vi "Go.vi"(9 "Timing Values":dbl[](array[numeric]), 10 "Control In":T1, 11 "CAD Dispense in":refnum<class "CAD Dispense.lvclass">) -> (2 "Control Out":T1, 3 "CAD Dispense Out":refnum<class "CAD Dispense.lvclass">)   [LabVIEW 2019, in "CAD Dispense.lvclass"]
uses:
  CAD Dispense.lvclass
  Controller/Controllers.ctl
  Controller/I-O/I-O.lvclass
  Controller/Dispenser/Dispenser.lvclass
  C:/Program Files (x86)/Aerotech/A3200/LabVIEW/2010/Bin/Aerotech.A3200.dll
  Program Files (x86)/Aerotech/A3200/LabVIEW/2010/Bin/Aerotech.A3200.dll
  CAD Dispense.lvclass/CAD Dispense.ctl
  Controller/Motion/A3200/A3200.lvclass
  Controller/Controller.lvclass
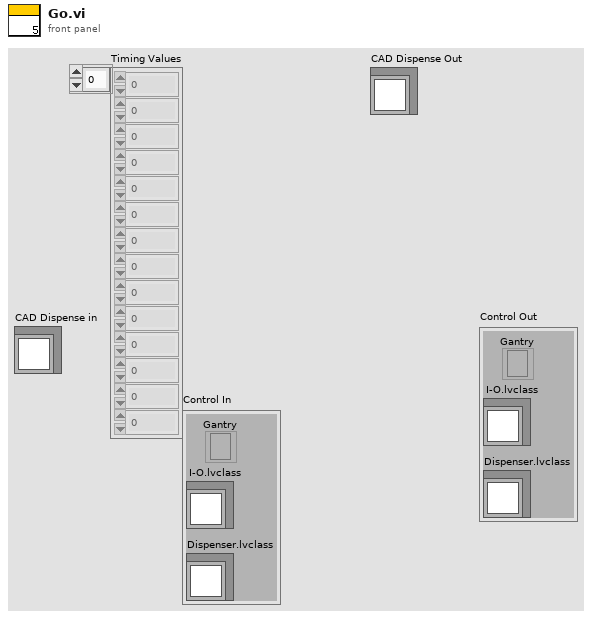
[diagram p1: front panel]
types:
  T1 = typedef "Controller.lvclass/Controllers.ctl" = cluster{"I-O.lvclass":refnum<class "I-O.lvclass">, "Dispenser.lvclass":refnum<class "Dispenser.lvclass">, "Gantry":refnum<k24>}
  T2 = cluster{"Motion":dbl[][], "Center":dbl[], "Circle?":bool, "CW/CCW":dbl}[]
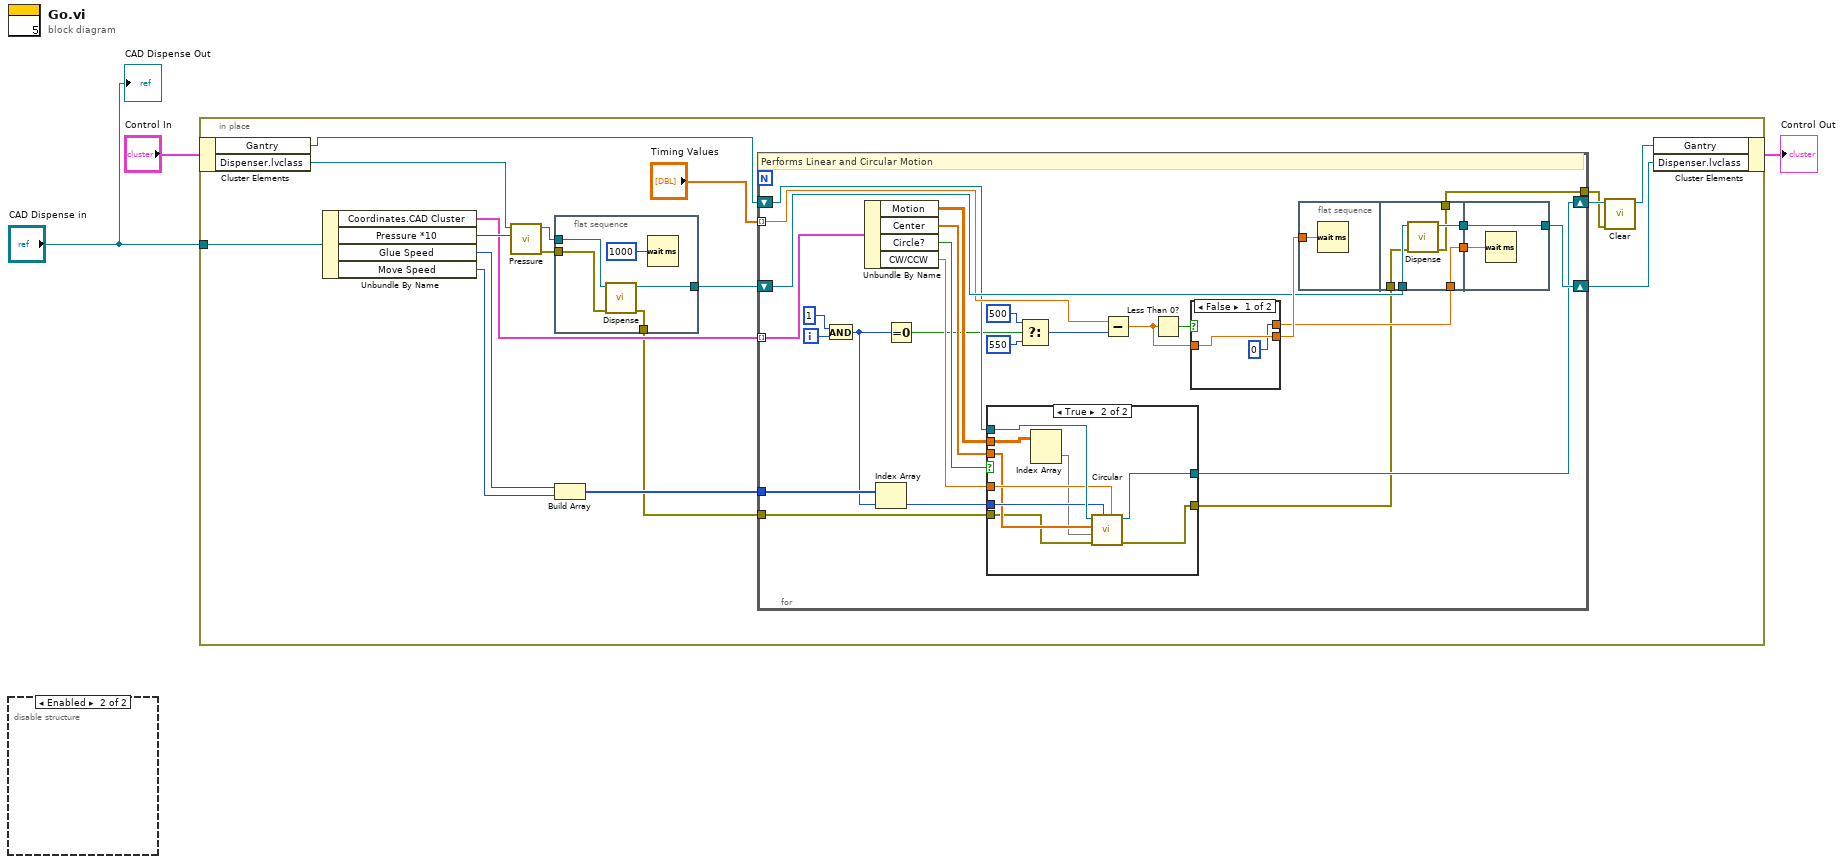
[diagram p0: block diagram]
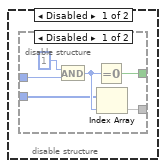
[diagram p2: hidden frame]
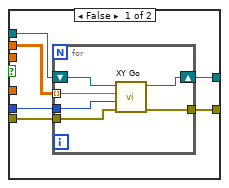
[diagram p4: hidden frame]
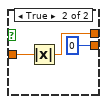
[diagram p5: hidden frame]
diagram:
  n1 = disable-structure shown="Enabled" {
    frame Disabled {
      n2 = disable-structure shown="Disabled" {
        disable-tunnel: [w8 _] -> _
        disable-tunnel: _ -> [w7 _]
        disable-tunnel: [w5 _] -> _
        disable-tunnel: _ -> [w4 _]
        frame Disabled {
          n3 = And(x=1, y=w7) -> (x .and. y?=w6:i32)
          n4 = Equal To 0?(x=w6) -> (x = 0?=w5:bool)
          n5 = Index Array(array=w4, index=w6) -> (element=w8)
        }
        frame Enabled {
        }
      }
    }
    frame Enabled {
    }
  }
  n6 = in-place {
    in-place-border: "CAD Dispense in" -> [w25]
    n7 = in-place-cluster #1("Control In") -> ("Gantry"=w19:refnum<k24>, "Dispenser.lvclass"=w16:refnum<class "Dispenser.lvclass">)
    n8 = Unbundle By Name(w25) -> ("Coordinates.CAD Cluster"=w12:T2, "Pressure *10"=w15:i64, "Glue Speed"=w23:i32, "Move Speed"=w22:i32)
    n9 = call-dynamic "Pressure.vi"("Pressure"=w15, "Dispenser in"=w16) -> ("error out"=w14:errorcluster, "Dispenser out"=w13:refnum<class "Dispenser.lvclass">)  [unwired: 8 in]
    n10 = flat-sequence {
      tunnel: [w29] -> w24
      tunnel: w14 -> [w28]
      tunnel: w13 -> [w30]
      tunnel: [w27] -> w11
      frame #0 {
        n11 = call-dynamic "Dispense.vi"("error in (no error)"=w28, "Dispenser in"=w30) -> ("error out"=w27:errorcluster, "Dispenser out"=w29:refnum<class "Dispenser.lvclass">)  [unwired: 8 in]
        n12 = Wait (ms)(milliseconds to wait=u32 1000) -> ()  [unwired: 1 out]
      }
    }
    n13 = Build Array(w23, w22) -> (w21:i32[])
    n14 = for {
      tunnel: w12 -> [w52] mode=indexing
      tunnel: "Timing Values" -> [w48] mode=indexing
      tunnel: w21 -> [w42]
      shift-right: [w45] -> w26
      shift-left: w24 -> [w54]
      shift-right: [w44] -> w18
      shift-left: w19 -> [w47]
      tunnel: w11 -> [w34]
      tunnel: [w32] -> w10
      i -> [w41]
      # "Performs Linear and Circular Motion"
      n15 = And(x=1, y=w41) -> (x .and. y?=w39:i32)
      n16 = Unbundle By Name(w52) -> ("Motion"=w51:dbl[][], "Center"=w50:dbl[], "Circle?"=w43:bool, "CW/CCW"=w46:dbl)
      n17 = Index Array(array=w42, index=w39) -> (element=w35:i32)
      n18 = Equal To 0?(x=w39) -> (x = 0?=w38:bool)
      n19 = case shown="True" w43 {
        tunnel: [w65 w78] -> w44
        tunnel: w46 -> [_ w76]
        tunnel: w51 -> [w63 w80]
        tunnel: w50 -> [_ w75]
        tunnel: w47 -> [w64 w79]
        tunnel: w35 -> [w62 w77]
        tunnel: w34 -> [w61 w73]
        tunnel: [w60 w72] -> w33
        frame False {
          n20 = for {
            tunnel: w63 -> [w69] mode=indexing
            shift-right: [w70] -> w65
            shift-left: w64 -> [w71]
            tunnel: w62 -> [w68]
            tunnel: w61 -> [w67]
            tunnel: [w66] -> w60
            n21 = call "XY Go.vi"("error in (no error)"=w67, "Speed"=w68, "XY"=w69, "Gantry In"=w71) -> ("error out"=w66:errorcluster, "Gantry Out"=w70:refnum<k24>)  [unwired: 6 in]
          }
        }
        frame True {
          n22 = Index Array(array=w80) -> (element=w74:dbl[])  [unwired: 2 in]
          n23 = call "Circular.vi"("Direction"=w76, "Speed"=w77, "error in (no error)"=w73, "XY End"=w74, "XY Center"=w75, "Gantry In"=w79) -> ("error out"=w72:errorcluster, "Gantry Out"=w78:refnum<k24>)  [unwired: 4 in]
        }
      }
      n24 = Select(t=500, s=w38, f=550) -> (s? t:f=w53:i32)
      n25 = Subtract(x=w48, y=w53) -> (x-y=w49:dbl)
      n26 = Less Than 0?(x=w49) -> (x < 0?=w59:bool)
      n27 = case shown="False" w59 {
        tunnel: [w90 u32 0 ("milliseconds to wait")] -> w58
        tunnel: w49 -> [w90 w93]
        tunnel: [u32 0 ("milliseconds to wait") w92] -> w57
        frame False {
        }
        frame True {
          n28 = Absolute Value(x=w93) -> (abs(x)=w92:dbl)
        }
      }
      n29 = flat-sequence {
        tunnel: w58 -> [w81]
        tunnel: w54 -> [w85]
        tunnel: [w86] -> w56
        tunnel: w57 -> [w86]
        tunnel: [w84] -> w55
        tunnel: w33 -> [w83]
        tunnel: [w82] -> w32
        tunnel: w56 -> [w88]
        tunnel: w55 -> [w87]
        tunnel: [w87] -> w45
        frame #0 {
          n30 = Wait (ms)(milliseconds to wait=w81) -> ()  [unwired: 1 out]
        }
        frame #1 {
          n31 = call-dynamic "Dispense.vi"("error in (no error)"=w83, "Dispenser in"=w85) -> ("error out"=w82:errorcluster, "Dispenser out"=w84:refnum<class "Dispenser.lvclass">)  [unwired: 8 in]
        }
        frame #2 {
          n32 = Wait (ms)(milliseconds to wait=w88) -> ()  [unwired: 1 out]
        }
      }
    }
    n33 = call "Clear.vi"("error in (no error)"=w10, "Gantry In"=w18) -> ("Gantry Out"=w17:refnum<k24>)  [unwired: 8 in, 1 out]
    n34 = in-place-cluster #1("Gantry"=w17, "Dispenser.lvclass"=w26) -> (→"Control Out":T1)
  }
  "CAD Dispense Out" <- "CAD Dispense in"
